vi "Test Grabber Tool Load.vi"() -> ()   [LabVIEW 2011]
uses:
  Config Manager Class/Type Definitions/Named Position.ctl
  GrabberTool Class.lvclass
  Gantry Class/Gantry Class.lvclass
panel:
  out "error out":errorcluster
  in  "Config Folder":path=path "C:/Users/Husker/Desktop/gantry/Config"
  in  "HOME?":bool
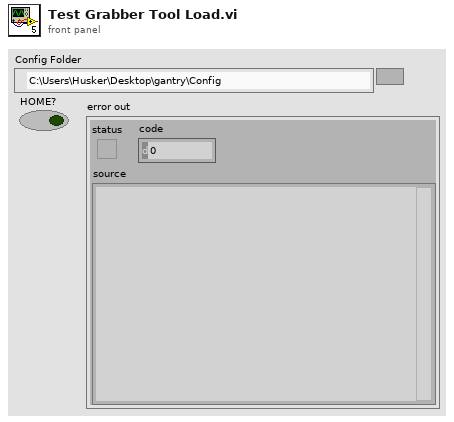
[diagram p1: front panel]
types:
  T1 = typedef "Named Position.ctl" = enum16{"home", "module_chuck_0", "module_chuck_1", "module_chuck_2", "module_chuck_3", "module_chuck_4", "glue_reservoir_chuck", "stamp_tool_chuck", "weight_tool_chuck", "needle_calibration", "tool_rack_pos_0_in", "tool_rack_pos_0_out", "tool_rack_pos_1_in", "tool_rack_pos_1_out", "tool_rack_pos_2_in", "tool_rack_pos_2_out", "front_load_position", "grabber_start_pos", "between_chuck_0_and_1", "between_chuck_2_and_3"}
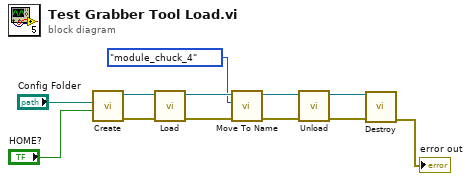
[diagram p0: block diagram]
diagram:
  n1 = call "Create.vi"("HOME?"="HOME?", "Config Folder"="Config Folder") -> ("error out"=w9:errorcluster, "Gantry out"=w10:refnum<class "Gantry Class.lvclass">)  [unwired: 8 in]
  n2 = call "Load.vi"("error in"=w9, "Gantry In"=w10) -> ("error out"=w7:errorcluster, "Grabber Tool out"=w8:refnum<class "GrabberTool Class.lvclass">)  [unwired: 8 in]
  n3 = call-dynamic "Move To Name.vi"("error in"=w7, "Destination"=Named_Position."module_chuck_4", "Gantry in"=w8) -> ("error out"=w5:errorcluster, "Gantry out"=w6:refnum<class "GrabberTool Class.lvclass">)  [unwired: 7 in]
  n4 = call "Unload.vi"("error in"=w5, "GrabberTool in"=w6) -> ("error out"=w3:errorcluster, "Gantry out"=w4:refnum<class "Gantry Class.lvclass">)  [unwired: 8 in]
  n5 = call "Destroy.vi"("error in"=w3, "Gantry Class in"=w4) -> ("error out"=→"error out":errorcluster)  [unwired: 9 in]
